vi "FTWLib-JSON-LibraryFilepath.vi"(8 "error in":errorcluster) -> (0 "error out":errorcluster, 2 "JSON Library Filepath":path)   [LabVIEW 2014]
uses:
  FTWLib-Jansson32.dll
  FTWLib-Jansson64.dll
  FTWLib-Jansson32.so
panel:
  # "Inputs"
  # "Outputs"
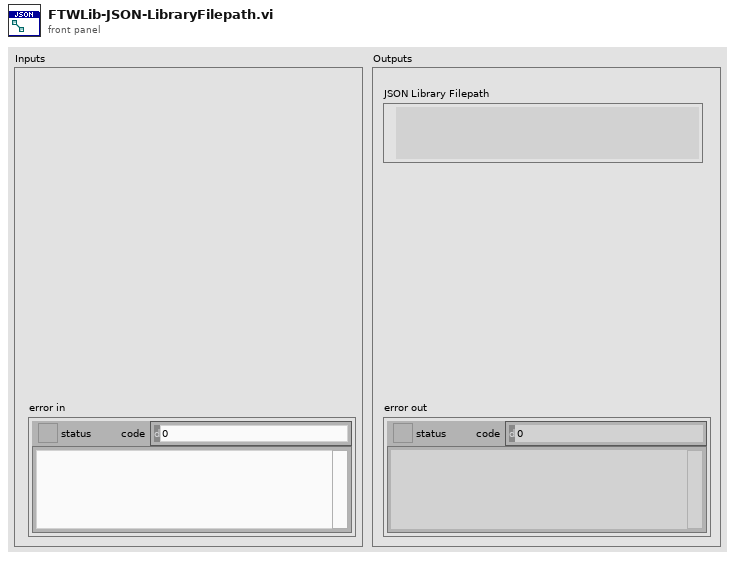
[diagram p1: front panel]
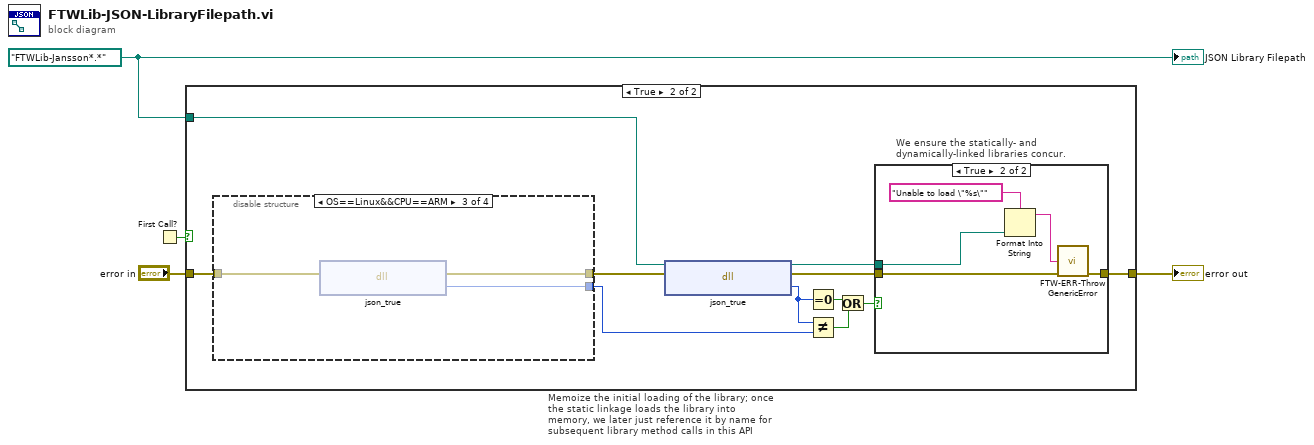
[diagram p0: block diagram]
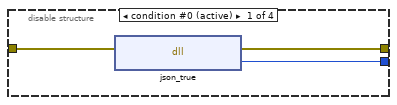
[diagram p4: hidden frame]
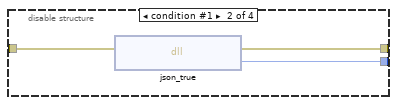
[diagram p5: hidden frame]
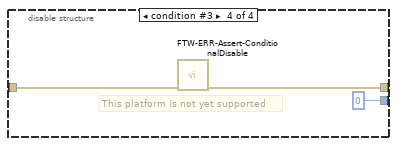
[diagram p6: hidden frame]
diagram:
  w1 = path "FTWLib-Jansson*.*"
  n1 = First Call?() -> (First Call?: T/F=w2:bool)
  n2 = case "Memoize the initial loading of the library; once the static linkage loads the library into memory, we later just reference it by name for subsequent library method calls in this API" shown="True" w2 {
    tunnel: "error in" -> [w5 w16]
    tunnel: [w5 w14] -> w3
    tunnel: w1 -> [_ w8]
    frame False {
    }
    frame True {
      n3 = disable-structure shown="OS==Linux&&CPU==ARM" {
        disable-tunnel: [w24 w27 w30 w32] -> w6
        disable-tunnel: w16 -> [w25 w28 w31 w33]
        disable-tunnel: [w23 w26 w29 i64 0 ("True Constant Pointer")] -> w15
        frame condition #0 (active) {
          n4 = dll-call lib="C:/Users/Jack/repo/ftw-master/ftw/lib/jansson/FTWLib-Jansson32.dll" fn="json_true" label="FTWLib-Jansson32.dll"(error in=w25) -> (error out=w24:errorcluster, "True Constant Pointer"=w23:i64)  [unwired: 2 in, 1 out]
        }
        frame condition #1 {
          n5 = dll-call lib="C:/Users/Jack/repo/ftw-master/ftw/lib/jansson/FTWLib-Jansson64.dll" fn="json_true" label="FTWLib-Jansson64.dll"(error in=w28) -> (error out=w27:errorcluster, "True Constant Pointer"=w26:i64)  [unwired: 2 in, 1 out]
        }
        frame condition #2 {
          n6 = dll-call lib="C:/Users/Jack/repo/ftw-master/ftw/lib/jansson/FTWLib-Jansson32.so" fn="json_true" label="FTWLib-Jansson32.so"(error in=w31) -> (error out=w30:errorcluster, "True Constant Pointer"=w29:i64)  [unwired: 2 in, 1 out]
        }
        frame condition #3 {
          # "This platform is not yet supported"
          n7 = call "FTW-ERR-Assert-ConditionalDisable.vi"("error in"=w33) -> ("error out"=w32:errorcluster)  [unwired: 14 in]
        }
      }
      n8 = dll-call lib="?" fn="json_true"(path in=w8, error in=w6) -> (path out=w7:path, error out=w13:errorcluster, "True Constant Pointer"=w12:i64)  [unwired: 1 in]
      n9 = Equal To 0?(x=w12) -> (x = 0?=w11:bool)
      n10 = Not Equal?(x=w12, y=w15) -> (x != y?=w10:bool)
      n11 = Or(x=w11, y=w10) -> (x .or. y?=w9:bool)
      n12 = case "We ensure the statically- and\ndynamically-linked libraries concur." shown="True" w9 {
        tunnel: w13 -> [w17 w22]
        tunnel: [w17 w21] -> w14
        tunnel: w7 -> [_ w18]
        frame False {
        }
        frame True {
          n13 = Format Into String(format string="Unable to load \"%s\"", w18) -> (resulting string=w20:string)  [unwired: 2 in, 1 out]
          n14 = call "FTW-ERR-ThrowGenericError.vi"("Error Message"=w20, "error in"=w22) -> ("error out"=w21:errorcluster)  [unwired: 13 in]
        }
      }
    }
  }
  "error out" <- w3
  "JSON Library Filepath" <- w1
